vi "Scan Status View.vi"(10 "User Events in":refnum<class "User Events.lvclass">) -> ()   [LabVIEW 2016, in "M1M3SupportEUI_Views.lvlib"]
uses:
  M1M3SupportEUI_Views.lvlib
  User Events/User Events.lvclass
  User Events/User Events.lvclass/User Events.ctl
  Typedefs/StateTypes.ctl
  Typedefs/M1M3SupportEUI_TypeDefs.lvlib
panel:
  out "State":string
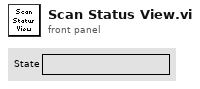
[diagram p1: front panel]
types:
  T1 = typedef "M1M3SupportEUI_TypeDefs.lvlib/Publish Data Events.ctl" = cluster{"State":refnum<user-event>, "ErrorCode":refnum<user-event>}
  T2 = cluster{"Event Registration Refnum":refnum<event-registration>, "Event Registration Refnum":refnum<event-registration>}
  T3 = typedef "M1M3SupportEUI_TypeDefs.lvlib/StateTypes.ctl" = enum16{"Offline State", "Fault State", "Standby State", "Disabled State", "Enabled State", "Wait For User Input State", "Test Actuator State"}
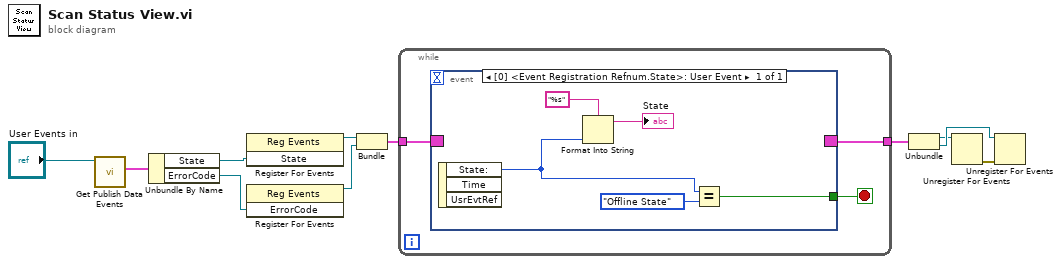
[diagram p0: block diagram]
diagram:
  n1 = call "Get Publish Data Events.vi"("UserEvents in"="User Events in") -> ("Publish Data Events"=w10:T1)  [unwired: 9 in, 1 out]
  n2 = Unbundle By Name(w10) -> ("State"=w9:refnum<user-event>, "ErrorCode"=w11:refnum<user-event>)
  n3 = register-events(w9) -> (reference out=w4:refnum<event-registration>)  [unwired: 2 in, 1 out]
  n4 = register-events(w11) -> (reference out=w5:refnum<event-registration>)  [unwired: 2 in, 1 out]
  n5 = Bundle("Event Registration Refnum"=w4, "Event Registration Refnum"=w5) -> (w3:T2)  [unwired: 1 in]
  n6 = while {
    tunnel: w3 -> [w14]
    tunnel: [w13] -> w2
    stop <- w12 stop-if-true
    n7 = event shown="[0] <Event Registration Refnum.State>: User Event" {
      selector: w14 -> [_]
      dyn-events: [_] -> w13
      timeout: _ -> [_]
      tunnel: [w18] -> w12
      event User Event {
        n8 = event-data() -> ("State:"=w15:T3)  [unwired: 1 in, 2 out]
        n9 = Format Into String(format string="%s", w15) -> (resulting string=→"State":string)  [unwired: 2 in, 1 out]
        n10 = Equal?(x=w15, y=StateTypes."Offline State") -> (x = y?=w18:bool)
      }
    }
  }
  n11 = Unbundle(w2) -> ("Event Registration Refnum"=w1:refnum<event-registration>, "Event Registration Refnum"=w6:refnum<event-registration>)
  n12 = Unregister For Events(event registration refnum=w1) -> (error out=w7:errorcluster)  [unwired: 1 in]
  n13 = Unregister For Events(event registration refnum=w6, error in=w7) -> ()  [unwired: 1 out]
